vi "Update Device Info.vi"(8 "error in":errorcluster, 11 "Manual Control in":refnum<class "Manual Control.lvclass">) -> (0 "error out":errorcluster, 3 "Manual Control out":refnum<class "Manual Control.lvclass">)   [LabVIEW 2018, in "Manual Control Actor.lvlib" / "Manual Control.lvclass"]
uses:
  Manual Control.lvclass
  C:/Users/Administrator/Desktop/2018LabVIEW EMS/EMS Generic Actor/EMS Generic/EMS Generic.lvclass
  C:/Program Files (x86)/National Instruments/LabVIEW 2018/vi.lib/ActorFramework/Actor/Actor.lvclass
  Manual Control.lvclass/Manual Control.ctl
  <vilib>/ActorFramework/Actor/Actor.lvclass/Actor.ctl
  EMS Generic Actor/EMS Generic/EMS Generic.lvclass/EMS Generic.ctl
  EMS Generic Actor/EMS Generic Messages/Return DER_Info Msg/Return DER_Info Msg.lvclass/Return DER_Info Msg.ctl
  <vilib>/ActorFramework/Message Enqueuer/Message Enqueuer.lvclass/Message Enqueuer.ctl
  <vilib>/ActorFramework/Message Enqueuer/Enqueue.vi
  EMS Generic Actor/EMS Generic Messages/Return DER_Info Msg/Return DER_Info Msg.lvclass
  C:/Program Files (x86)/National Instruments/LabVIEW 2018/vi.lib/ActorFramework/Message/Message.lvclass
  <vilib>/ActorFramework/Message Priority Queue/Priority Enqueue.vi
  <vilib>/ActorFramework/Actor/Actor.lvclass
  EMS Generic Actor/EMS Generic/EMS Generic.lvclass
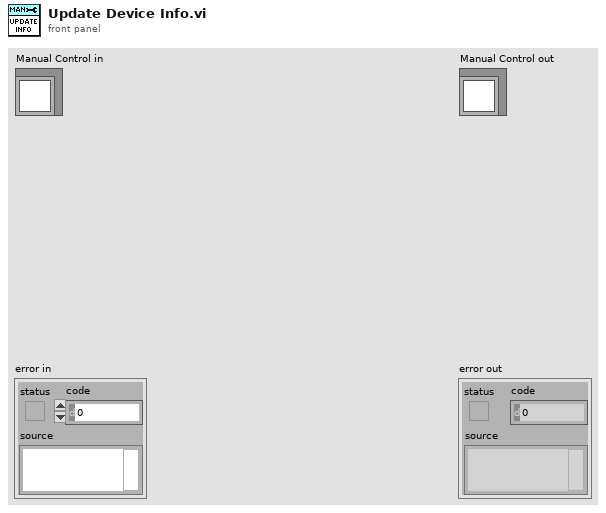
[diagram p1: front panel]
types:
  T1 = typedef "CSEISMIC DDS.lvlib/CSEISMIC DDS.lvclass/DeviceID.ctl" = string
  T2 = typedef "CSEISMIC DDS.lvlib/CSEISMIC DDS.lvclass/DER_Info.ctl" = cluster{"DeviceID":T1, "LineConfig":u8[], "NominalVoltage(V)":dbl, "PowerRating(kVA)":dbl, "VFControl":bool, "PControl":bool, "QControl":bool, "PFControl":bool, "PVControl":bool, "Droop":bool, "DroopConfigurable":bool, "Unbalanced":bool}
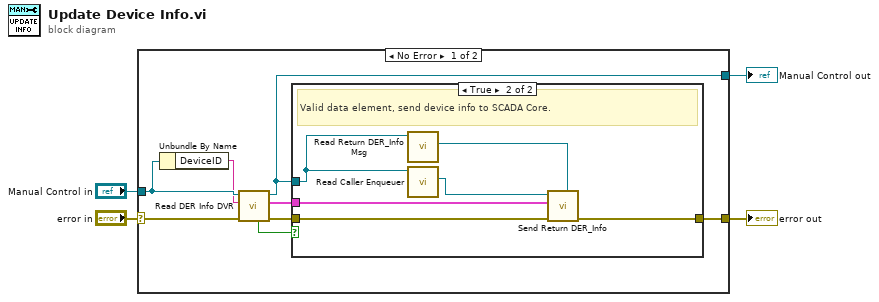
[diagram p0: block diagram]
diagram:
  n1 = case shown="No Error" "error in" {
    selector: "error in" -> [w10 w21]
    tunnel: [w6 w21] -> w3
    tunnel: [w9 w20] -> w1
    tunnel: "Manual Control in" -> [w12 w20]
    frame No Error {
      n2 = Unbundle By Name(w12) -> ("DeviceID"=w11:T1)
      n3 = call "Read DER Info DVR.vi"("error in"=w10, "DeviceID"=w11, "EMS Generic in"=w12) -> ("error out"=w7:errorcluster, "DER_Info"=w8:T2, "EMS Generic out"=w9:refnum<class "Manual Control.lvclass">, "valid?"=w5:bool)  [unwired: 5 in]
      n4 = case shown="True" w5 {
        tunnel: w9 -> [_ w15]
        tunnel: w8 -> [_ w16]
        tunnel: w7 -> [w13 w18]
        tunnel: [w13 w17] -> w6
        frame False {
          # "#TODO Should this be an error?"
          # "#TODO Should update status on Master Controller Core"
          # "No info data available for specified device"
        }
        frame True {
          # "Valid data element, send device info to SCADA Core."
          n5 = call "Read Return DER_Info Msg.vi"("EMS Generic in"=w15) -> ("Return DER_Info Msg"=w14:refnum<class "Return DER_Info Msg.lvclass">)  [unwired: 9 in, 1 out]
          n6 = call <vilib>:"Read Caller Enqueuer.vi"("Actor"=w15) -> ("Caller Enqueuer"=w19:refnum<class "Message Enqueuer.lvclass">)  [unwired: 10 in]
          n7 = call "Send Return DER_Info.vi"("Message Type"=w14, "error in (no error)"=w18, "DER_Info"=w16, "Message Enqueuer"=w19) -> ("error out"=w17:errorcluster)  [unwired: 6 in, 1 out]
        }
      }
    }
    frame Error {
    }
  }
  "error out" <- w3
  "Manual Control out" <- w1
